vi "8-Axis Roadshow Demo KNR-IPAD.vi"() -> ()   [LabVIEW 2013]
uses:
  Typedef/Typedef_Motor_Message.ctl
  EMC API/EMC_Typedef_Motor_Parameters.ctl
  Functional_Global/Typedef_Message_Queue_Action.ctl
  Functional_Global/Typedef_FPGA_Interface_Action.ctl
  Globals/Global Stop.vi
  <vilib>/Motion/Express/_s/nimc.ex.clearFaults.clearFaults.axis.vi
  <vilib>/Motion/Express/_s/nimc.ex.power.power.axis.vi
  <vilib>/Motion/Express/_s/nimc.ex.resetPosition.resetPosition.axis.vi
  Globals/Default Motor Parameters.vi
  <vilib>/Motion/Express/_s/nimc.ex.read.readTrajectoryData.axis.vi
  <vilib>/Motion/BlockNode/FB.NIMotion.xnode
  support/Message Queue/Message Queue.lvlib
  <vilib>/NI_Real-Time Target Support.lvlib
panel:
  in  "# whole revs":dbl=3.0 format="%#_13g"
  in  "Stop all motors":bool
  in  "Max delay (ms)":u32=1000
  in  "Motion Parameters (Min)":T1={"position"=-10000.0, "velocity"=-10000.0, "acceleration"=50000.0, "deceleration"=50000.0, "accel. jerk"=800000.0, "decel. jerk"=800000.0}
  in  "Motion Parameters (Max)":T1={"position"=10000.0, "velocity"=10000.0, "acceleration"=100000.0, "deceleration"=100000.0, "accel. jerk"=1000000.0, "decel. jerk"=1000000.0}
  in  "Command Array":string[](array[string])=["ABS Pos Move", "REL Pos Move", "Velocity Move"]
  out "Command":T2={"Axis"="", "Motion Parameters"={"position"=1000.0, "velocity"=1000.0, "acceleration"=10000.0, "deceleration"=10000.0, "accel. jerk"=10000.0, "decel. jerk"=10000.0}}
  out "Message":string
  out "# elements in queue":i32
  out "error out":errorcluster
  out "Axis Positions":T3(graph)
  out "Axis Velocities":T3(graph)
  out "Array":dbl[](array[knob]) scale=0.0..1600.0
  in  "stop":bool
  # "This example demonstrates how to set up an multi-axis SW architecture using SoftMotion.  You can have state machines that \"produce\" the motion commands, and the consumer will then digest them one at a time.\n\nIn this example, 3 producer loops generate random motion commands at random times (within 1000ms each iteration.) This VI is also meant as a stress test to see if the SM engine is robust enough for complex sequences of motion commands."
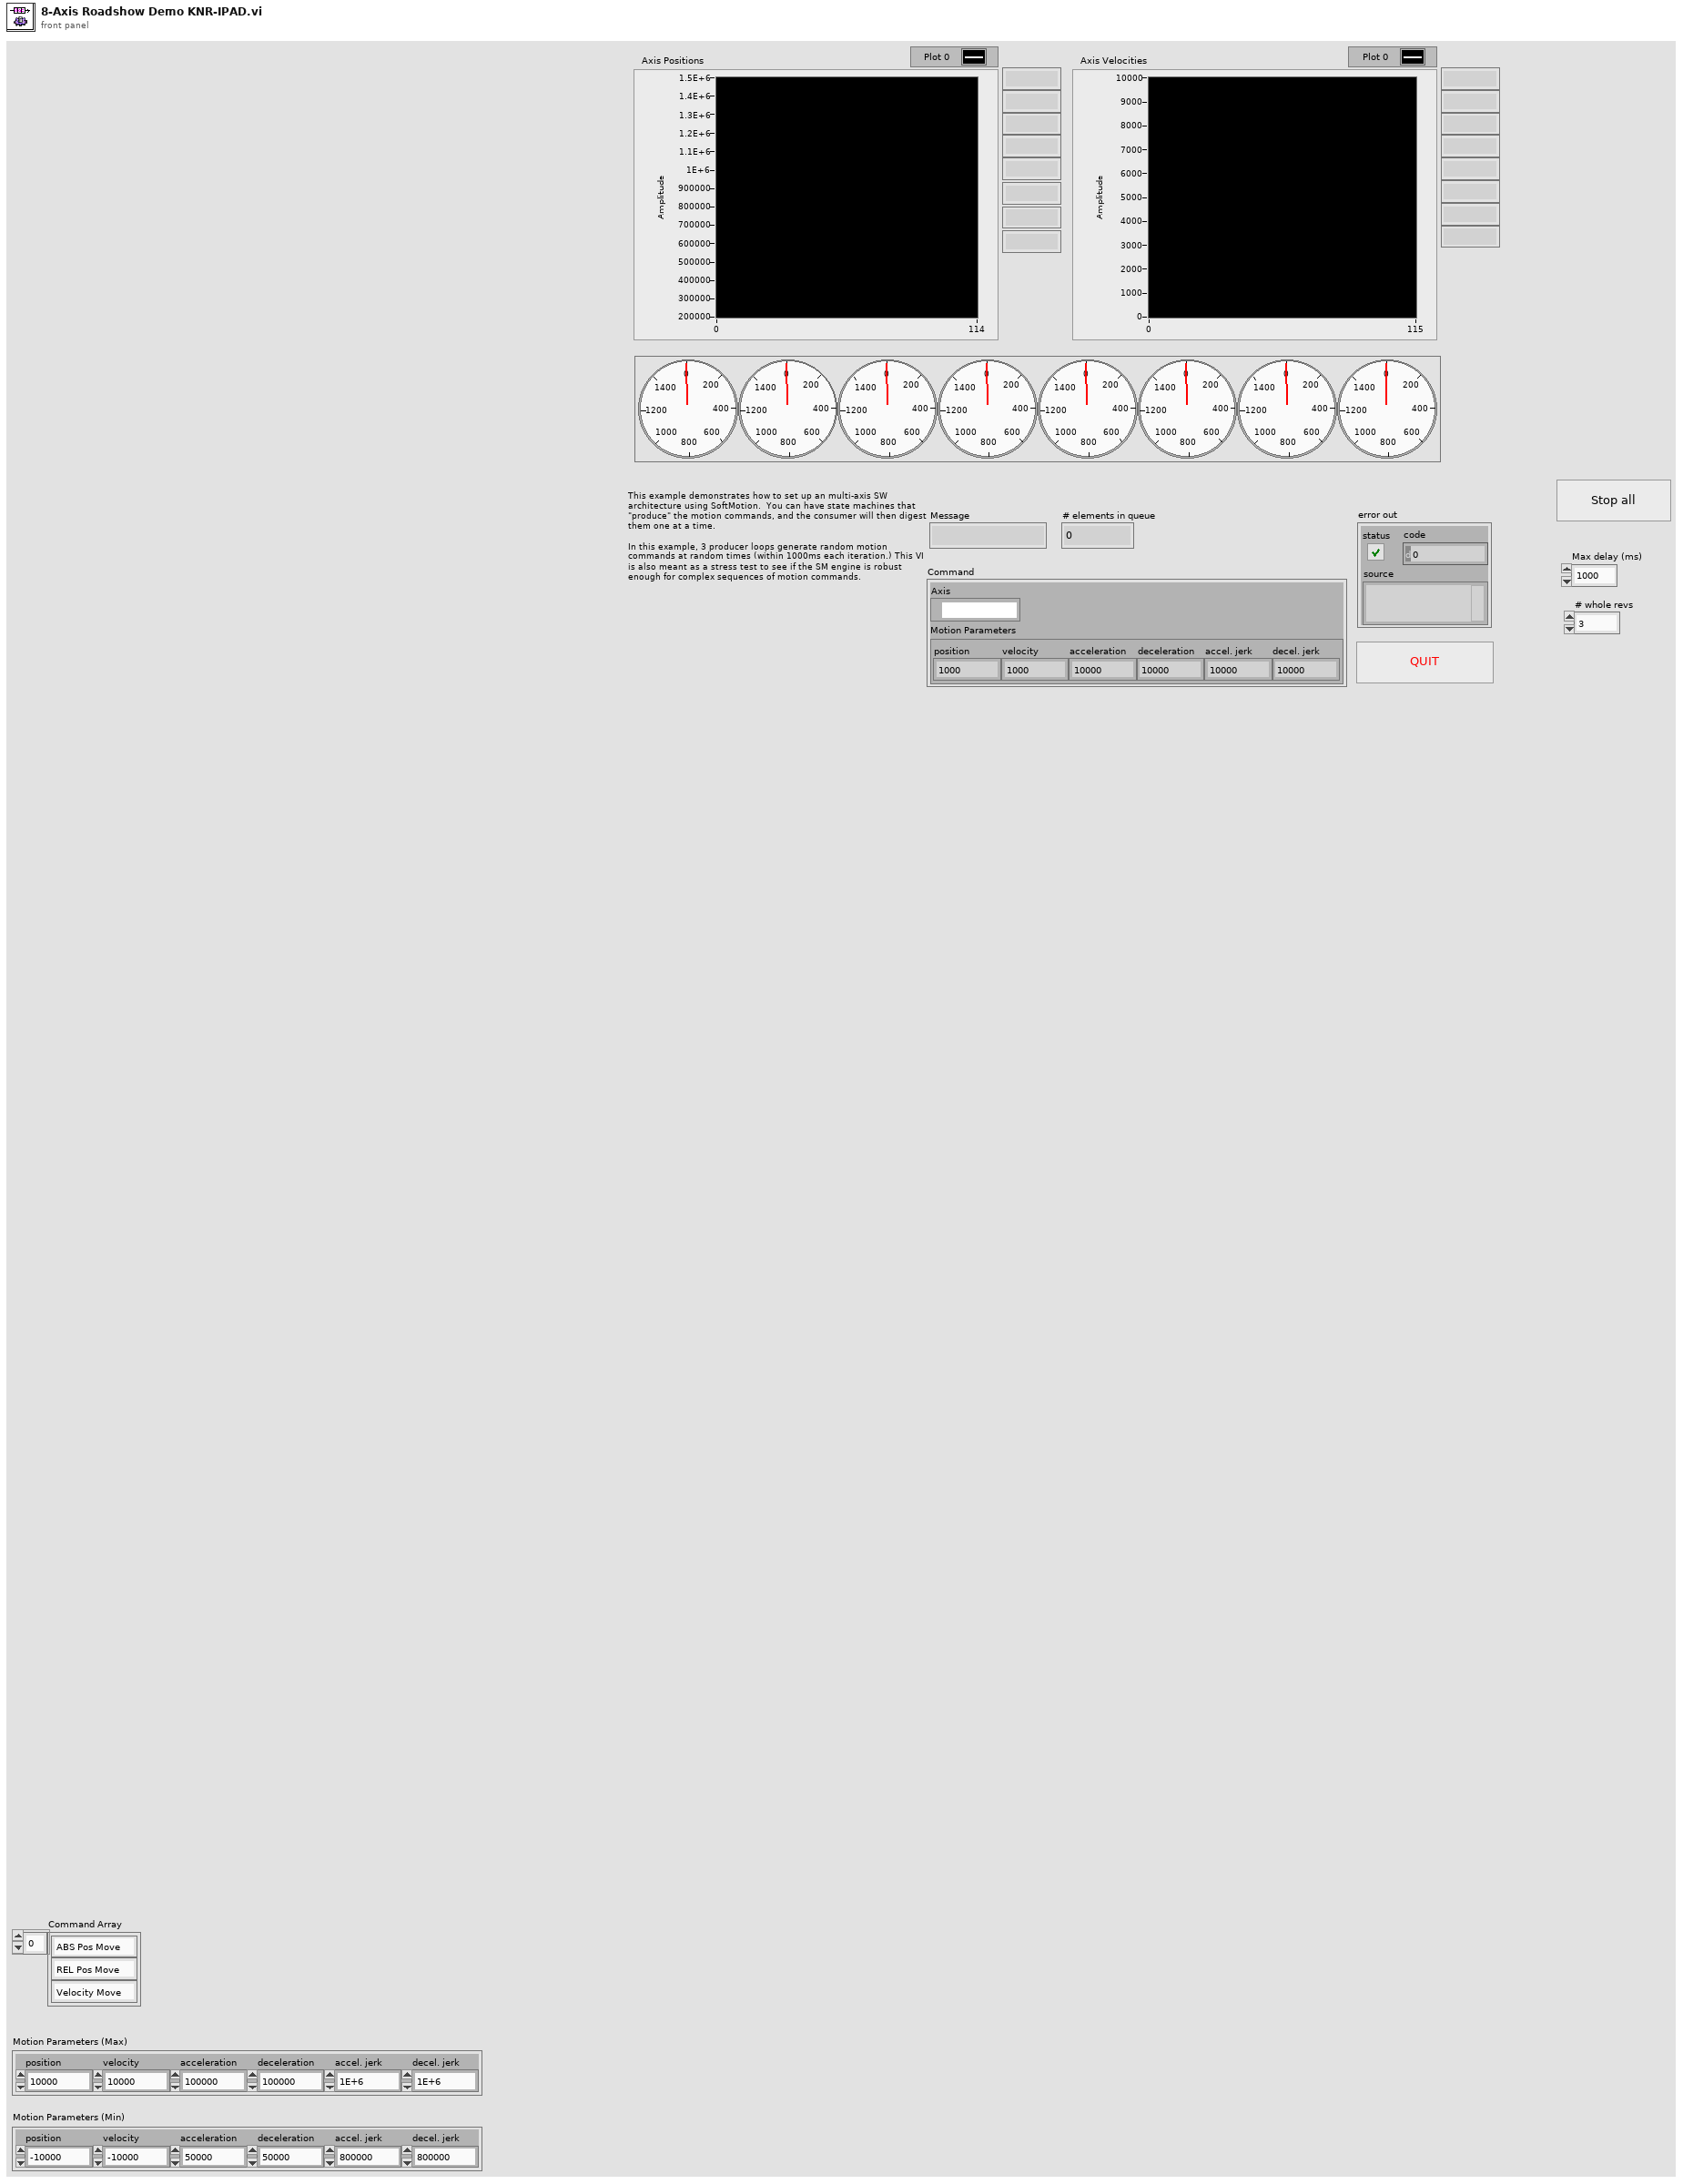
[diagram p1: front panel]
types:
  T1 = typedef "EMC_Typedef_Motor_Parameters.ctl" = cluster{"position":dbl, "velocity":dbl, "acceleration":dbl, "deceleration":dbl, "accel. jerk":dbl, "decel. jerk":dbl}
  T2 = typedef "Typedef_Motor_Message.ctl" = cluster{"Axis":refnum<k21>, "Motion Parameters":T1}
  T3 = cluster{"[0]":dbl, "[1]":dbl, "[2]":dbl, "[3]":dbl, "[4]":dbl, "[5]":dbl, "[6]":dbl, "[7]":dbl}
  T4 = typedef "Typedef_Message_Queue_Action.ctl" = enum16{"Init MQueue", "Get MQueue Ref", "Close MQueue"}
  T5 = typedef "Typedef_FPGA_Interface_Action.ctl" = enum16{"Initialize FPGA", "Get FPGA Reference", "Close FPGA"}
  T6 = typedef "Message Queue.lvlib/Message Cluster.ctl" = cluster{"Message":string, "Message Data":variant}
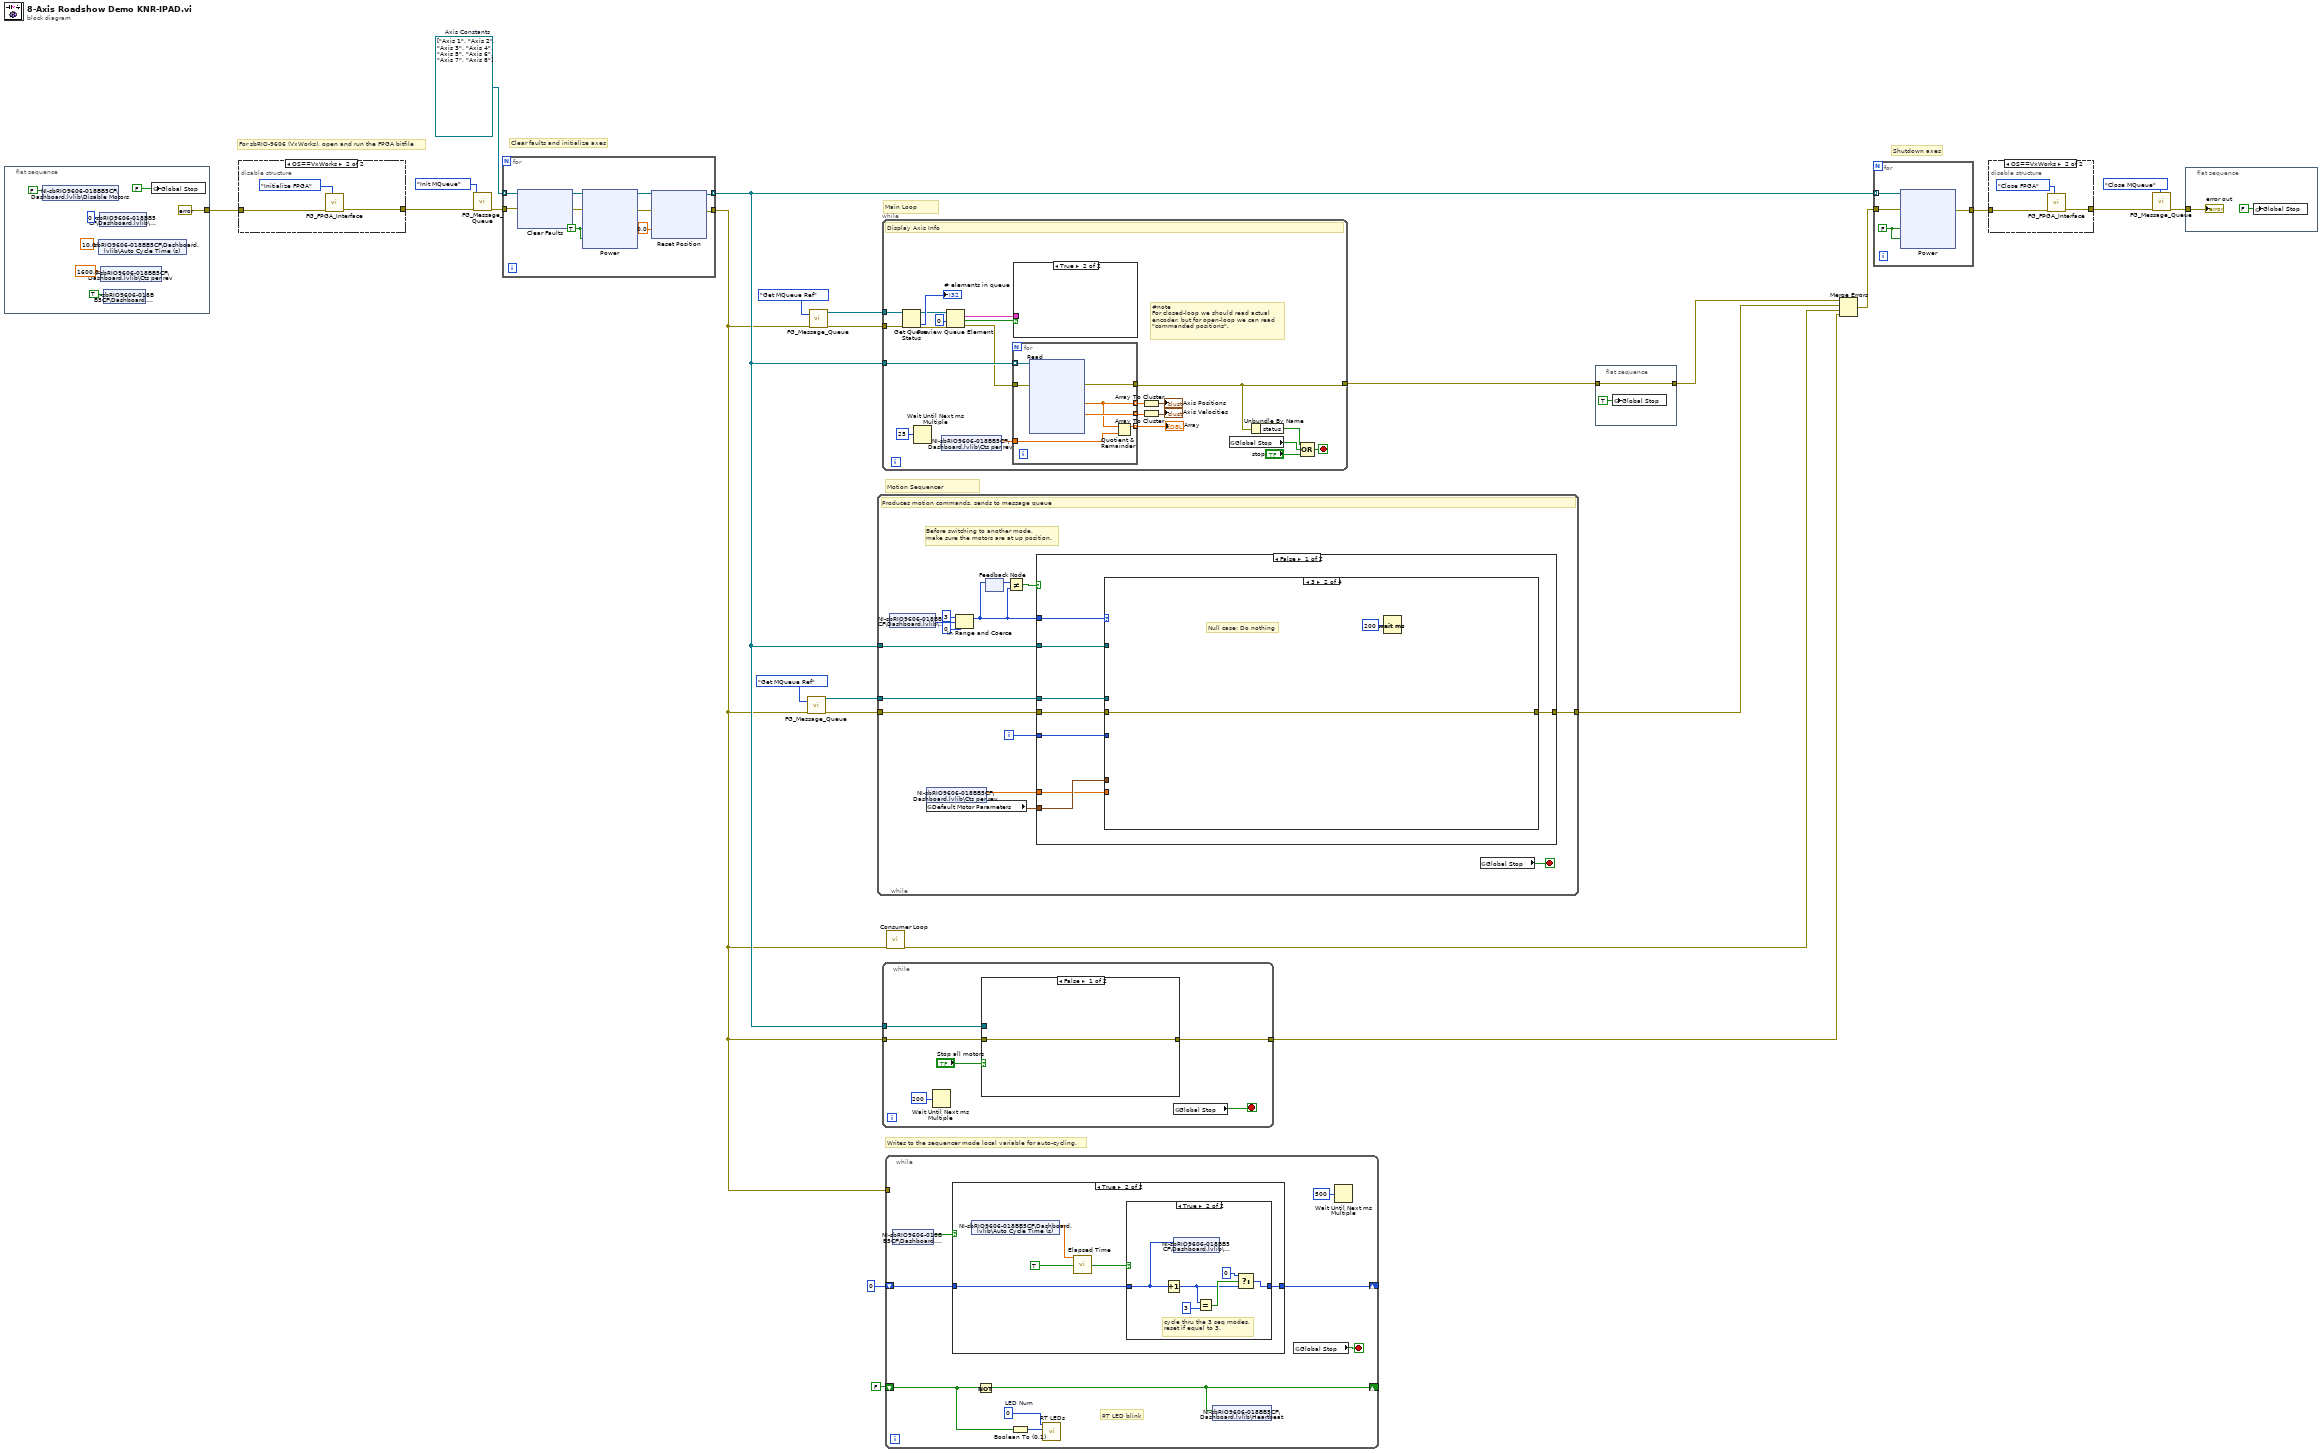
[diagram p0: block diagram]
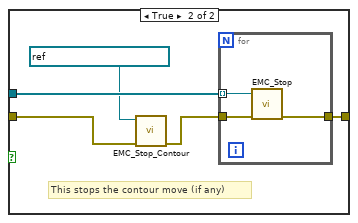
[diagram p4: hidden frame]
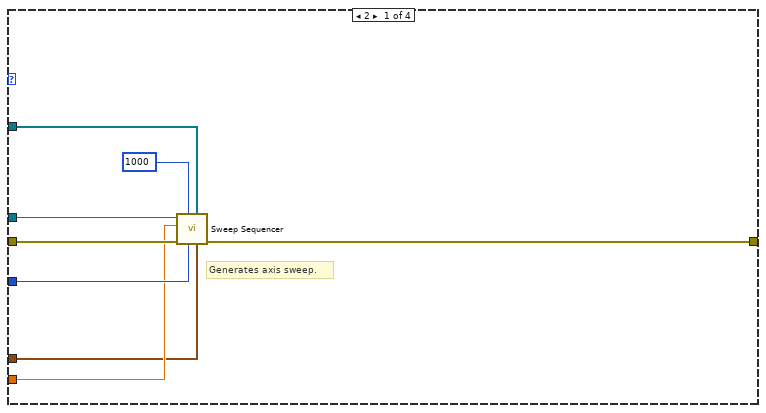
[diagram p5: hidden frame]
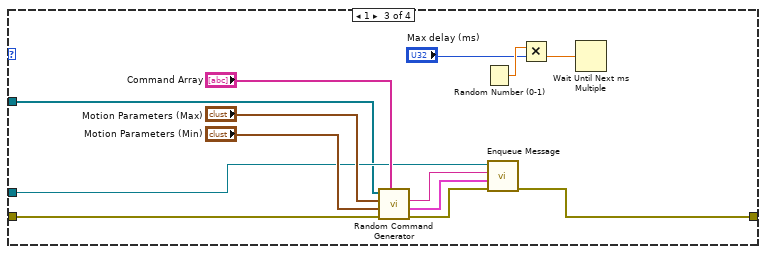
[diagram p6: hidden frame]
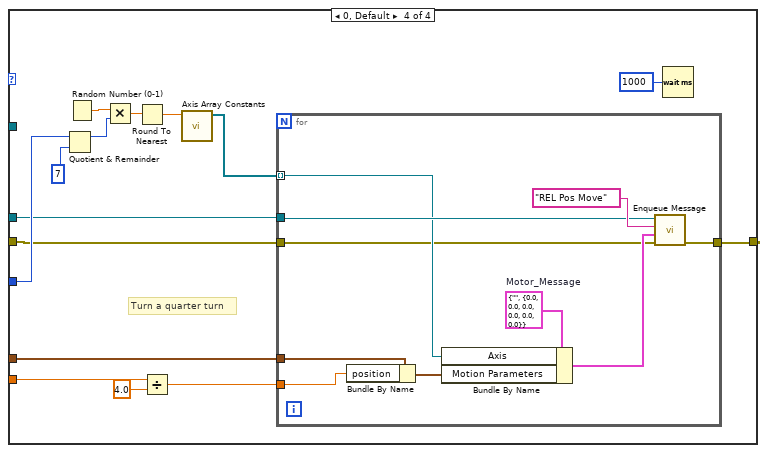
[diagram p7: hidden frame]
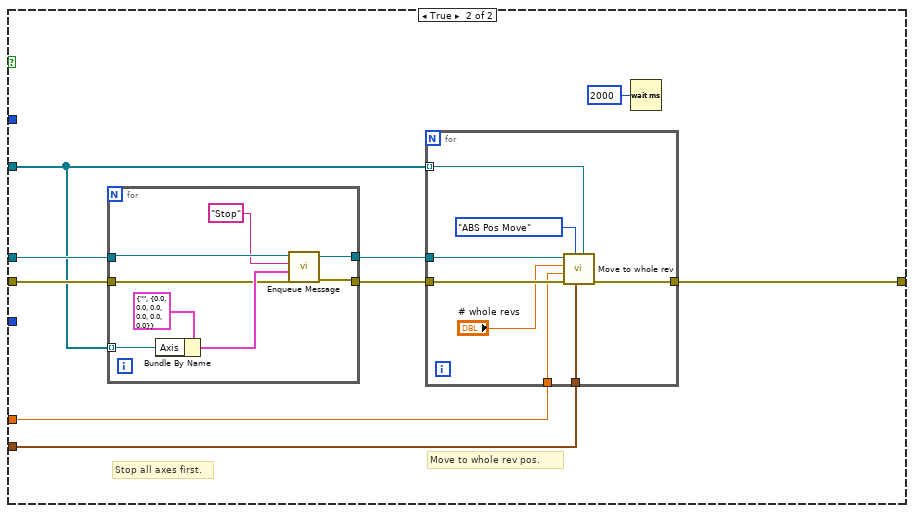
[diagram p8: hidden frame]
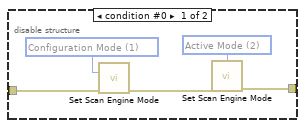
[diagram p10: hidden frame]
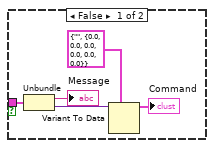
[diagram p11: hidden frame]
diagram:
  w24 = refnum<k21>[] ["Axis 1", "Axis 2", "Axis 3", "Axis 4", "Axis 5", "Axis 6", "Axis 7", "Axis 8"]  # Axis Constants
  # "Writes to the sequencer mode local variable for auto-cycling."
  # "Motion Sequencer"
  # "For sbRIO-9606 (VxWorks), open and run the FPGA bitfile"
  # "Shutdown axes"
  # "Main Loop"
  # "Clear faults and initialize axes"
  n1 = flat-sequence {
    tunnel: [errorcluster {"status"=FALSE, "code"=0, "source"=""} ("error in (no error)")] -> w25
    frame #0 {
      n2 = shared-variable "NI-sbRIO9606-018BB5CF\\Dashboard.lvlib\\Disable Motors"(FALSE ("Disable Motors")) -> ()  [unwired: 1 in, 1 out]
      n3 = shared-variable "NI-sbRIO9606-018BB5CF\\Dashboard.lvlib\\Auto Cycle Time (s)"(10.0 ("Auto Cycle Time (s)")) -> ()  [unwired: 1 in, 1 out]
      n4 = shared-variable "NI-sbRIO9606-018BB5CF\\Dashboard.lvlib\\Mode"(u16 0 ("Mode")) -> ()  [unwired: 1 in, 1 out]
      n5 = shared-variable "NI-sbRIO9606-018BB5CF\\Dashboard.lvlib\\Cts per rev"(1600.0 ("Cts per rev")) -> ()  [unwired: 1 in, 1 out]
      n6 = shared-variable "NI-sbRIO9606-018BB5CF\\Dashboard.lvlib\\Auto"(TRUE ("Auto")) -> ()  [unwired: 1 in, 1 out]
      n7 = global write "Global Stop.vi" "Global Stop"(FALSE ("stop")) -> ()
    }
  }
  n8 = disable-structure shown="OS==VxWorks" {
    disable-tunnel: [w37 w38] -> w20
    disable-tunnel: w25 -> [w36 w39]
    frame condition #0 {
      w33 = 1 items=["Configuration Mode"=1, "Active Mode"=2] ("mode (Active Mode)")
      w34 = 2 items=["Configuration Mode"=1, "Active Mode"=2] ("mode (Active Mode)")
      n9 = call <vilib>:"Set Scan Engine Mode.vi"("mode (Active Mode)"=w33, "error in (no error)"=w36) -> ("error out"=w35:errorcluster)  [unwired: 13 in]
      n10 = call <vilib>:"Set Scan Engine Mode.vi"("mode (Active Mode)"=w34, "error in (no error)"=w35) -> ("error out"=w37:errorcluster)  [unwired: 13 in]
    }
    frame condition #1 (active) {
      n11 = call "FG_FPGA_Interface.vi"("Action"=Typedef_FPGA_Interface_Action."Initialize FPGA", "error in"=w39) -> ("error out"=w38:errorcluster)  [unwired: 9 in]
    }
  }
  n12 = call "FG_Message_Queue.vi"("Action"=Typedef_Message_Queue_Action."Init MQueue", "error in"=w20) -> ("error out"=w19:errorcluster)  [unwired: 8 in, 1 out]
  n13 = for {
    tunnel: [w47] -> w3
    tunnel: [w45] -> w5 mode=indexing
    tunnel: w19 -> [w41]
    tunnel: w24 -> [w44] mode=indexing
    w50 = TRUE ("enable axis")
    n14 = xnode ("Clear Faults")("resource"=w44, "error in"=w41) -> ("resource out"=w43:refnum<k21>, "error out"=w42:errorcluster)
    n15 = xnode ("Power")("enable axis"=w50, "enable drive"=w50, "resource"=w43, "error in"=w42) -> ("resource out"=w46:refnum<k21>, "error out"=w48:errorcluster)
    n16 = xnode ("Reset Position")("position"=0.0, "resource"=w46, "error in"=w48) -> ("resource out"=w45:refnum<k21>, "error out"=w47:errorcluster)
  }
  n17 = call "FG_Message_Queue.vi"("Action"=Typedef_Message_Queue_Action."Get MQueue Ref", "error in"=w3) -> ("error out"=w8:errorcluster, "Message Queue"=w7:refnum<queue>)  [unwired: 8 in]
  n18 = call "FG_Message_Queue.vi"("Action"=Typedef_Message_Queue_Action."Get MQueue Ref", "error in"=w3) -> ("error out"=w11:errorcluster, "Message Queue"=w12:refnum<queue>)  [unwired: 8 in]
  n19 = while {
    tunnel: w5 -> [w80]
    tunnel: w8 -> [w82]
    tunnel: w7 -> [w81]
    tunnel: [w78] -> w6
    i -> [w79]
    stop <- w83 stop-if-true
    # "Before switching to another mode,\nmake sure the motors are at up position."
    # "Produces motion commands, sends to message queue"
    n20 = shared-variable "NI-sbRIO9606-018BB5CF\\Dashboard.lvlib\\Mode"() -> (w74:u16)  [unwired: 1 in, 1 out]
    n21 = shared-variable "NI-sbRIO9606-018BB5CF\\Dashboard.lvlib\\Cts per rev"() -> (w70:dbl)  [unwired: 1 in, 1 out]
    n22 = global read "Default Motor Parameters.vi" "Default Motor Parameters"() -> (w75:T1)
    n23 = In Range and Coerce(upper limit=u16 3, x=w74, lower limit=u16 0) -> (coerced(x)=w71:u16)  [unwired: 1 out]
    n24 = feedback-in #1(w71) -> ()
    n25 = feedback #1() -> (w77:u16)  [unwired: 1 in]
    n26 = Not Equal?(x=w77, y=w71) -> (x != y?=w76:bool)
    n27 = case shown="False" w76 {
      tunnel: w82 -> [w91 w145]
      tunnel: w81 -> [w90 w146]
      tunnel: w80 -> [w89 w142]
      tunnel: w79 -> [w88 _]
      tunnel: [w87 w148] -> w78
      tunnel: w71 -> [w86 _]
      tunnel: w75 -> [w85 w141]
      tunnel: w70 -> [w84 w140]
      frame False {
        n28 = case shown="3" w86 {
          tunnel: w91 -> [w99 w101 w108 w127]
          tunnel: w90 -> [w97 _ w107 w125]
          tunnel: w89 -> [w95 _ w106 _]
          tunnel: w88 -> [w98 _ _ w128]
          tunnel: [w96 w101 w103 w126] -> w87
          tunnel: w85 -> [w92 _ _ w120]
          tunnel: w84 -> [w93 _ _ w119]
          frame 2 {
            # "Generates axis sweep."
            n29 = call "Sweep Sequencer.vi"("Default Motor Parameters"=w92, "Axis Array"=w95, "Loop counter in"=w98, "Max delay (ms)"=u32 1000, "error in (no error)"=w99, "cts per rev"=w93, "Message Queue"=w97) -> ("error out"=w96:errorcluster)  [unwired: 4 in]
          }
          frame 3 {
            # "Null case: Do nothing"
            n30 = Wait (ms)(milliseconds to wait=u32 200) -> ()  [unwired: 1 out]
          }
          frame 1 {
            n31 = call "Random Command Generator.vi"("Command Array"="Command Array", "error in (no error)"=w108, "Motion Parameters (Min)"="Motion Parameters (Min)", "Motion Parameters (Max)"="Motion Parameters (Max)", "Axis Resources"=w106) -> ("error out"=w109:errorcluster, "Motor_Message"=w111:T2, "Command Out"=w110:string)  [unwired: 4 in]
            n32 = Random Number (0-1)() -> (number: 0 to 1=w104:dbl)
            n33 = call "Enqueue Message.vi"("error in (no error)"=w109, "Message Data"=w111, "Message"=w110, "Message Queue"=w107) -> ("error out"=w103:errorcluster)  [unwired: 6 in, 1 out]
            n34 = Multiply(x=w104, y="Max delay (ms)") -> (x*y=w105:dbl)
            n35 = Wait Until Next ms Multiple(millisecond multiple=w105) -> ()  [unwired: 1 out]
          }
          frame 0, Default {
            # "Turn a quarter turn"
            n36 = Quotient & Remainder(x=w128, y=7) -> (x-y*floor(x/y)=w122:i32)  [unwired: 1 out]
            n37 = Random Number (0-1)() -> (number: 0 to 1=w123:dbl)
            n38 = Multiply(x=w123, y=w122) -> (x*y=w121:dbl)
            n39 = Round To Nearest(number=w121) -> (nearest integer value=w115:dbl)
            n40 = Divide(x=w119, y=4.0) -> (x/y=w117:dbl)
            n41 = call "Axis Array Constants.vi"("Numeric"=w115) -> ("Axis Constants"=w116:refnum<k21>[])  [unwired: 10 in]
            n42 = for {
              tunnel: w116 -> [w134] mode=indexing
              tunnel: w127 -> [w133]
              tunnel: [w132] -> w126
              tunnel: w117 -> [w135]
              tunnel: w125 -> [w136]
              tunnel: w120 -> [w130]
              w139 = T2 {"Axis"="", "Motion Parameters"={"position"=0.0, "velocity"=0.0, "acceleration"=0.0, "deceleration"=0.0, "accel. jerk"=0.0, "decel. jerk"=0.0}}  # Motor_Message
              n43 = Bundle By Name(cluster=w130, "position"=w135) -> (w131:T1)
              n44 = Bundle By Name(cluster=w139, "Axis"=w134, "Motion Parameters"=w131) -> (w138:T2)
              n45 = call "Enqueue Message.vi"("error in (no error)"=w133, "Message Data"=w138, "Message"="REL Pos Move", "Message Queue"=w136) -> ("error out"=w132:errorcluster)  [unwired: 6 in, 1 out]
            }
            n46 = Wait (ms)(milliseconds to wait=u32 1000) -> ()  [unwired: 1 out]
          }
        }
      }
      frame True {
        # "Move to whole rev pos."
        # "Stop all axes first."
        n47 = for {
          tunnel: w146 -> [w156]
          tunnel: w145 -> [w150]
          tunnel: [w149] -> w144
          tunnel: [w154] -> w143
          tunnel: w142 -> [w151] mode=indexing
          n48 = Bundle By Name(cluster=T2 {"Axis"="", "Motion Parameters"={"position"=0.0, "velocity"=0.0, "acceleration"=0.0, "deceleration"=0.0, "accel. jerk"=0.0, "decel. jerk"=0.0}} ("Motor_Message"), "Axis"=w151) -> (w152:T2)
          n49 = call "Enqueue Message.vi"("error in (no error)"=w150, "Message Data"=w152, "Message"="Stop", "Message Queue"=w156) -> ("error out"=w149:errorcluster, "dup Message Queue"=w154:refnum<queue>)  [unwired: 6 in]
        }
        n50 = for {
          tunnel: w142 -> [w160] mode=indexing
          tunnel: w144 -> [w164]
          tunnel: [w163] -> w148
          tunnel: w143 -> [w162]
          tunnel: w141 -> [w159]
          tunnel: w140 -> [w158]
          n51 = call "Move to whole rev.vi"("resource in"=w160, "Default Motor Parameters"=w159, "Mode"=enum16{"ABS Pos Move", "REL Pos Move"}."ABS Pos Move", "error in (no error)"=w164, "cts per rev"=w158, "# whole revs"="# whole revs", "Queue in"=w162) -> ("error out"=w163:errorcluster)  [unwired: 3 in, 1 out]
        }
        n52 = Wait (ms)(milliseconds to wait=u32 2000) -> ()  [unwired: 1 out]
      }
    }
    n53 = global read "Global Stop.vi" "Global Stop"() -> (w83:bool)
  }
  n54 = while {
    tunnel: w11 -> [w175]
    tunnel: w5 -> [w184]
    tunnel: [w169] -> w22
    tunnel: w12 -> [w177]
    stop <- w178 stop-if-true
    # "#note \nFor closed-loop we should read actual \nencoder, but for open-loop we can read\n\"commanded positions\"."
    # "Display Axis Info"
    n55 = Get Queue Status(queue=w177, error in (no error)=w175) -> (queue out=w171:refnum<queue>, error out=w173:errorcluster, # elements in queue=→"# elements in queue":i32)  [unwired: 1 in, 5 out]
    n56 = Wait Until Next ms Multiple(millisecond multiple=u32 25) -> ()  [unwired: 1 out]
    n57 = shared-variable "NI-sbRIO9606-018BB5CF\\Dashboard.lvlib\\Cts per rev"() -> (w167:dbl)  [unwired: 1 in, 1 out]
    n58 = Preview Queue Element(queue=w171, timeout in ms (-1)=0, error in (no error)=w173) -> (element=w170:T6, timed out?=w168:bool, error out=w172:errorcluster)  [unwired: 1 out]
    n59 = for {
      tunnel: [w198] -> w169
      tunnel: [w194] -> w166 mode=indexing
      tunnel: [w197] -> w165 mode=indexing
      tunnel: w172 -> [w196]
      tunnel: w184 -> [w195] mode=indexing
      tunnel: [w193] -> w183 mode=indexing
      tunnel: w167 -> [w192]
      n60 = xnode ("Read")("resource"=w195, "error in"=w196) -> ("commanded position"=w194:dbl, "commanded vel."=w197:dbl, "error out"=w198:errorcluster)  [unwired: 2 out]
      n61 = Quotient & Remainder(x=w194, y=w192) -> (x-y*floor(x/y)=w193:dbl)  [unwired: 1 out]
    }
    "Array" <- w183
    n62 = case shown="True" w168 {
      tunnel: w170 -> [w191 _]
      frame False {
        n63 = Unbundle(w191) -> ("Message"=→"Message":string, "Message Data"=w188:variant)
        n64 = Variant To Data(type=T2 {"Axis"="", "Motion Parameters"={"position"=0.0, "velocity"=0.0, "acceleration"=0.0, "deceleration"=0.0, "accel. jerk"=0.0, "decel. jerk"=0.0}} ("Motor_Message"), Variant=w188) -> (data=→"Command":T2)  [unwired: 1 in, 1 out]
      }
      frame True {
      }
    }
    n65 = Array To Cluster(array=w165) -> (cluster=→"Axis Velocities":T3)
    n66 = Array To Cluster(array=w166) -> (cluster=→"Axis Positions":T3)
    n67 = global read "Global Stop.vi" "Global Stop"() -> (w179:bool)
    n68 = Unbundle By Name(w169) -> ("status"=w180:bool)
    n69 = Compound Arithmetic op=OR(w180, w179, "stop") -> (w178:bool)
  }
  n70 = while {
    tunnel: w3 -> [w211]
    tunnel: w5 -> [w209]
    tunnel: [w208] -> w4
    stop <- w207 stop-if-true
    n71 = Wait Until Next ms Multiple(millisecond multiple=u32 200) -> ()  [unwired: 1 out]
    n72 = case shown="False" "Stop all motors" {
      tunnel: w211 -> [w212 w215]
      tunnel: [w212 w217] -> w208
      tunnel: w209 -> [_ w216]
      frame False {
      }
      frame True {
        # "This stops the contour move (if any)"
        n73 = call "EMC_Stop_Contour.vi"("error in (no error)"=w215, "coordinate"=refnum<k21> "Coordinate Space 1") -> ("error out"=w213:errorcluster)  [unwired: 9 in]
        n74 = for {
          tunnel: w213 -> [w220]
          tunnel: w216 -> [w218] mode=indexing
          tunnel: [w219] -> w217
          n75 = call "EMC_Stop.vi"("error in (no error)"=w220, "axis"=w218) -> ("error out"=w219:errorcluster)  [unwired: 8 in, 1 out]
        }
      }
    }
    n76 = global read "Global Stop.vi" "Global Stop"() -> (w207:bool)
  }
  n77 = while {
    tunnel: w3 -> [_]
    shift-right: [w226] -> _
    shift-left: 0 -> [w227]
    shift-right: [w221] -> _
    shift-left: FALSE -> [w222]
    stop <- w229 stop-if-true
    w224 = 0  # LED Num
    # "RT LED blink"
    n78 = shared-variable "NI-sbRIO9606-018BB5CF\\Dashboard.lvlib\\Auto"() -> (w225:bool)  [unwired: 1 in, 1 out]
    n79 = case shown="True" w225 {
      tunnel: w227 -> [w230 w234]
      tunnel: [w230 w233] -> w226
      frame False {
      }
      frame True {
        n80 = shared-variable "NI-sbRIO9606-018BB5CF\\Dashboard.lvlib\\Auto Cycle Time (s)"() -> (w231:dbl)  [unwired: 1 in, 1 out]
        n81 = call "Elapsed Time"("Time Target (s)"=w231, "Auto Reset"=TRUE) -> ("Time has Elapsed"=w235:bool)  [unwired: 10 in, 7 out]
        n82 = case shown="True" w235 {
          tunnel: w234 -> [w236 w237]
          tunnel: [w236 w238] -> w233
          frame False {
          }
          frame True {
            # "cycle thru the 3 seq modes,\nreset if equal to 3."
            n83 = Increment(x=w237) -> (x+1=w240:i32)
            n84 = shared-variable "NI-sbRIO9606-018BB5CF\\Dashboard.lvlib\\Mode"(w237) -> ()  [unwired: 1 in, 1 out]
            n85 = Equal?(x=w240, y=3) -> (x = y?=w241:bool)
            n86 = Select(t=0, s=w241, f=w240) -> (s? t:f=w238:i32)
          }
        }
      }
    }
    n87 = Not(x=w222) -> (.not. x?=w221:bool)
    n88 = Boolean To (0,1)(Boolean=w222) -> (0, 1=w223:i16)
    n89 = call <vilib>:"RT LEDs.vi"("State"=w223, "LED Num"=w224) -> ()  [unwired: 4 in, 2 out]
    n90 = shared-variable "NI-sbRIO9606-018BB5CF\\Dashboard.lvlib\\Heartbeat"(w221) -> ()  [unwired: 1 in, 1 out]
    n91 = global read "Global Stop.vi" "Global Stop"() -> (w229:bool)
    n92 = Wait Until Next ms Multiple(millisecond multiple=u32 500) -> ()  [unwired: 1 out]
  }
  n93 = call "Consumer Loop.vi"("error in (no error)"=w3) -> ("error out"=w10:errorcluster)  [unwired: 10 in]
  n94 = flat-sequence {
    tunnel: w22 -> [w243]
    tunnel: [w243] -> w14
    frame #0 {
      n95 = global write "Global Stop.vi" "Global Stop"(TRUE ("stop")) -> ()
    }
  }
  n96 = Merge Errors(w14, w6, w10, w4) -> (w18:errorcluster)
  n97 = for {
    tunnel: w5 -> [w248] mode=indexing
    tunnel: [w246] -> w23
    tunnel: w18 -> [w245]
    w247 = FALSE ("enable axis")
    n98 = xnode ("Power")("enable axis"=w247, "enable drive"=w247, "resource"=w248, "error in"=w245) -> ("error out"=w246:errorcluster)  [unwired: 1 out]
  }
  n99 = disable-structure shown="OS==VxWorks" {
    disable-tunnel: [w259 w260] -> w16
    disable-tunnel: w23 -> [w259 w261]
    frame condition #0 {
    }
    frame condition #1 (active) {
      n100 = call "FG_FPGA_Interface.vi"("Action"=Typedef_FPGA_Interface_Action."Close FPGA", "error in"=w261) -> ("error out"=w260:errorcluster)  [unwired: 9 in]
    }
  }
  n101 = call "FG_Message_Queue.vi"("Action"=Typedef_Message_Queue_Action."Close MQueue", "error in"=w16) -> ("error out"=w15:errorcluster)  [unwired: 8 in, 1 out]
  n102 = flat-sequence {
    tunnel: w15 -> [w263]
    frame #0 {
      n103 = global write "Global Stop.vi" "Global Stop"(FALSE ("stop")) -> ()
      "error out" <- w263
    }
  }
